vi "SetNewGame.vi"(8 "error in (no error)":errorcluster, 10 "NewGame":refnum<class "Game.lvclass">, 11 "Game in":refnum<class "Game.lvclass">) -> (0 "error out":errorcluster, 3 "Game out":refnum<class "Game.lvclass">)   [LabVIEW 2019, in "RT_Game.lvlib" / "Game.lvclass"]
uses:
  Game.lvclass
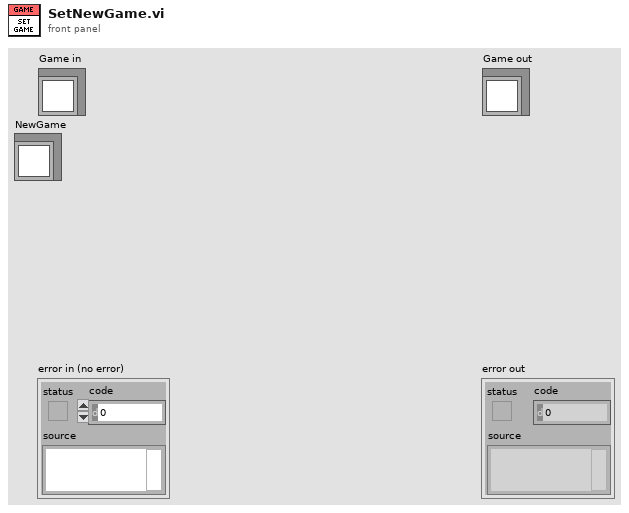
[diagram p1: front panel]
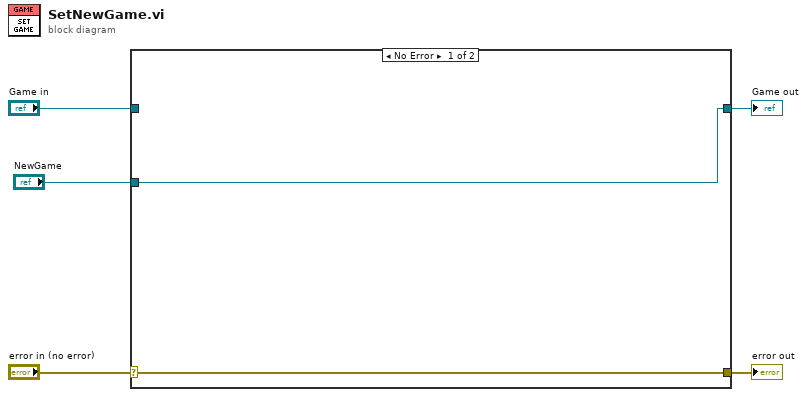
[diagram p0: block diagram]
diagram:
  n1 = case shown="No Error" "error in (no error)" {
    selector: "error in (no error)" -> [w7 w9]
    tunnel: [w7 w9] -> w4
    tunnel: [w6 w8] -> w2
    tunnel: "Game in" -> [_ w8]
    tunnel: "NewGame" -> [w6 _]
    frame No Error {
    }
    frame Error {
    }
  }
  "error out" <- w4
  "Game out" <- w2
